vi "check if data changed.vi"(2 "Data":variant, 4 "Allow Report on Time? (F)":bool) -> (5 "Data Changed?":bool)   [LabVIEW 2020, in "Template.lvlib" / "Template.lvclass"]
doc: "Checks if the data has changed. If so, returns True"
uses:
  Template.lvclass
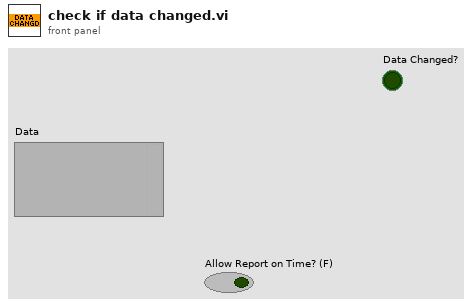
[diagram p1: front panel]
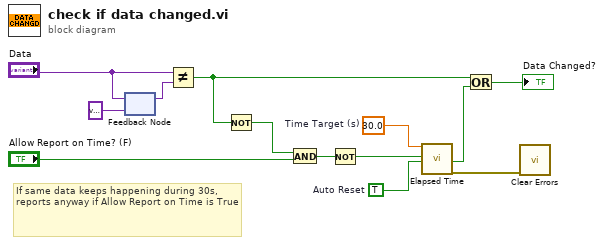
[diagram p0: block diagram]
diagram:
  w9 = TRUE  # Auto Reset
  w10 = 30.0  # Time Target (s)
  # "If same data keeps happening during 30s, reports anyway if Allow Report on Time is True"
  n1 = feedback #1(variant ("Data")) -> (w12:variant)
  n2 = feedback-in #1("Data") -> ()
  n3 = Not Equal?(x="Data", y=w12) -> (x != y?=w2:bool)
  n4 = Not(x=w2) -> (.not. x?=w1:bool)
  n5 = And(x=w1, y="Allow Report on Time? (F)") -> (x .and. y?=w3:bool)
  n6 = Not(x=w3) -> (.not. x?=w5:bool)
  n7 = call "Elapsed Time"("Time Target (s)"=w10, "Reset"=w5, "Auto Reset"=w9) -> ("Time has Elapsed"=w7:bool, "error out"=w4:errorcluster)  [unwired: 9 in, 6 out]
  n8 = Or(x=w2, y=w7) -> (x .or. y?=→"Data Changed?":bool)
  n9 = call <vilib>:"Clear Errors.vi"("error in (no error)"=w4) -> ()  [unwired: 5 in, 2 out]
